vi "Result.Parse STD OUT Text, Create Result Data.vi"(4 "UUTDir":path, 6 "Prefix":string, 7 "Category":string, 8 "Version Name":string, 9 "Error Code":i32, 10 "Task Name":string, 11 "StdOut":string) -> (0 "Error":errorcluster, 1 "SW Ver":T4[](array[typedef]), 2 "Numeric":T5[](array[typedef]) {"Status" items=["LOG", "PASS", "FAIL", "ERROR"]}, 3 "Attr":T2[](array[typedef]) {"Status" items=["LOG", "PASS", "FAIL", "ERROR"]}, 5 "Data Files":T1[](array[typedef]))   [LabVIEW 2018]
uses:
  Result.Numeric.ctl
  Result.Limit Type.ctl
  Result.Measurement and Attribute Item Status.ctl
  Result XML/TestResult.SW Item.ctl
  Result.Attribute.ctl
  Reports/Report.Result FileDataObject.ctl
  Errors/Error.Error Code List.ctl
  <vilib>/KATE/Files/File Utils.lvlib
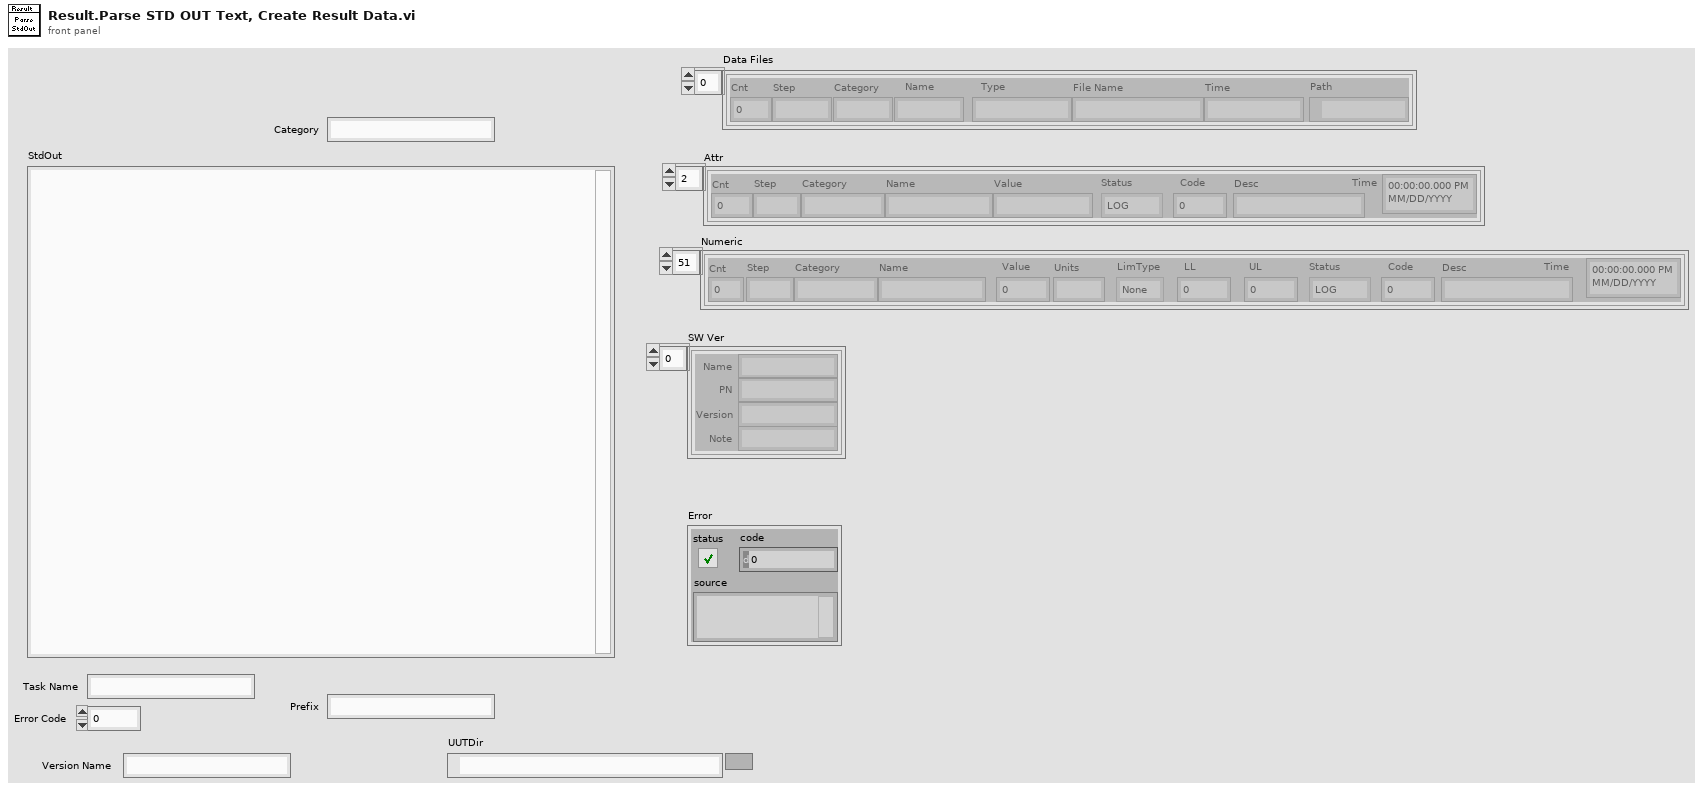
[diagram p1: front panel]
types:
  T1 = typedef "Report.Result FileDataObject.ctl" = cluster{"Cnt":i32, "Step":string, "Category":string, "Name":string, "Type":string, "File Name":string, "Time":string, "Path":path}
  T2 = typedef "Result.Attribute.ctl" = cluster{"Cnt":i32, "Step":string, "Category":string, "Name":string, "Value":string, "Status":T3, "Code":i32, "Desc":string, "Time":timestamp}
  T3 = typedef "Result.Measurement and Attribute Item Status.ctl" = i32
  T4 = typedef "TestResult.SW Item.ctl" = cluster{"Name":string, "PN":string, "Version":string, "Note":string}
  T5 = typedef "Result.Numeric.ctl" = cluster{"Cnt":i32, "Step":string, "Category":string, "Name":string, "Value":dbl, "Units":string, "LimType":T6, "LL":dbl, "UL":dbl, "Status":T3, "Code":i32, "Desc":string, "Time":timestamp}
  T6 = typedef "Result.Limit Type.ctl" = enum16{"None", "EQ", "NE", "GT", "LT", "GE", "LE", "GTLT", "GELE", "GELT", "GTLE", "LTGT", "LEGE", "LEGT", "LTGE", "Contains", "NotContains"}
  T7 = cluster{"Attr":T2[], "Numeric":T5[], "SW Ver":T4[], "Error":errorcluster, "Data Files":T1[]}
  T8 = typedef "Error.Error Code List.ctl" = i32
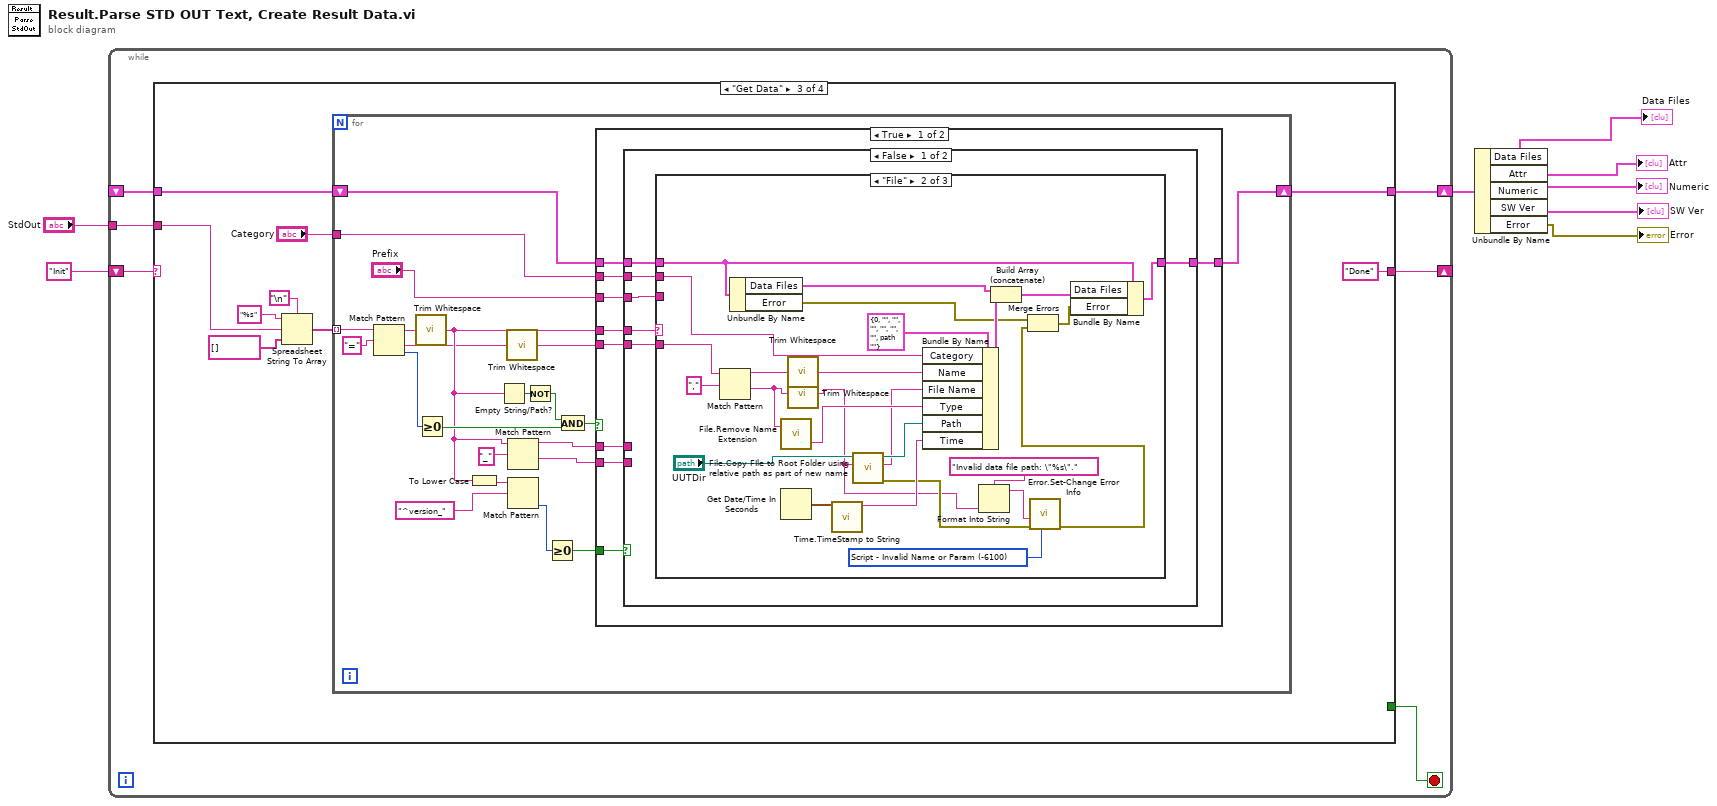
[diagram p0: block diagram]
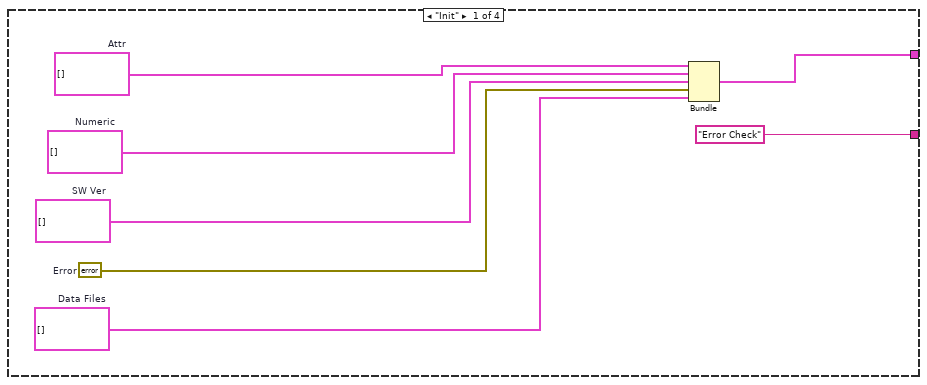
[diagram p2: hidden frame]
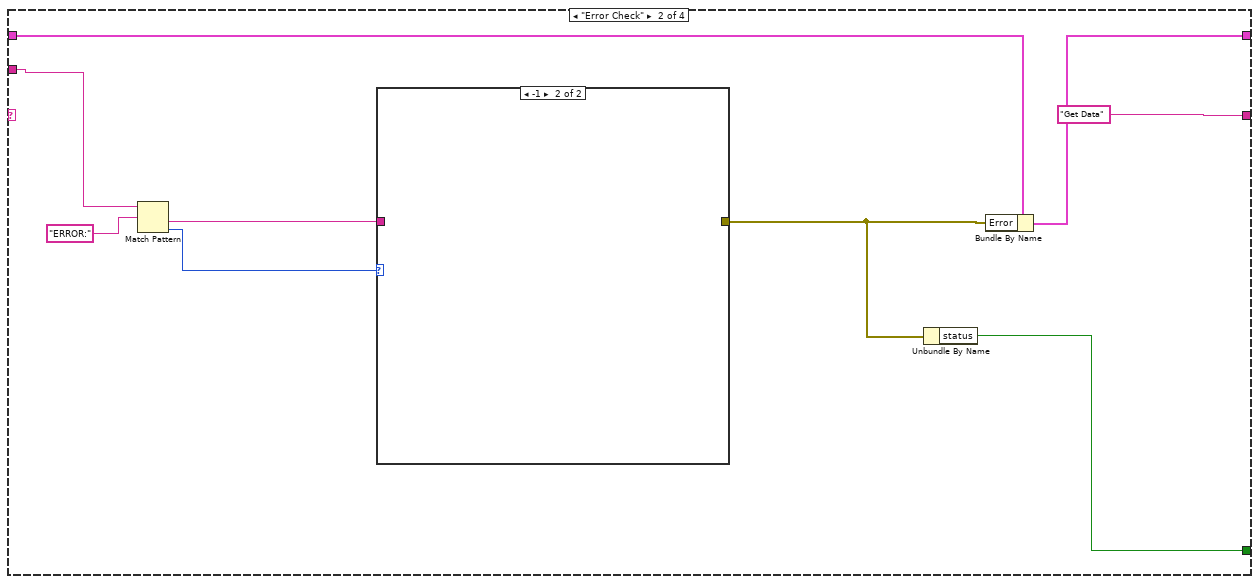
[diagram p3: hidden frame]
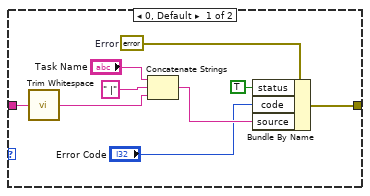
[diagram p4: hidden frame]
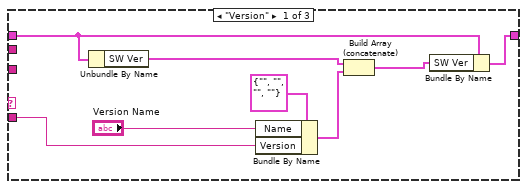
[diagram p5: hidden frame]
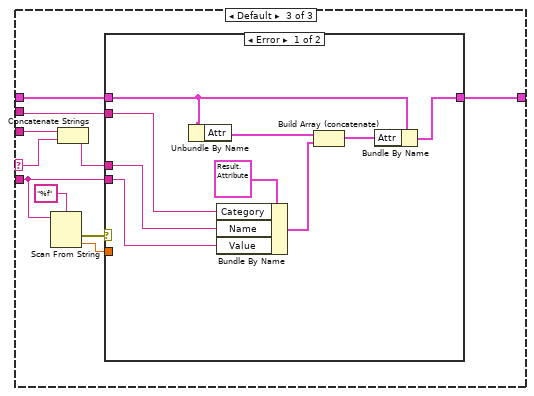
[diagram p6: hidden frame]
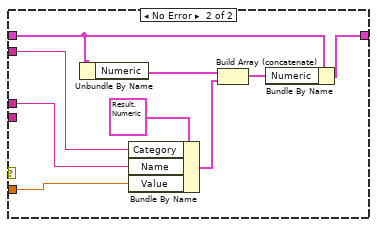
[diagram p7: hidden frame]
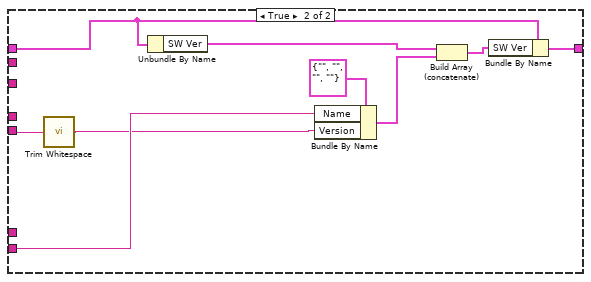
[diagram p8: hidden frame]
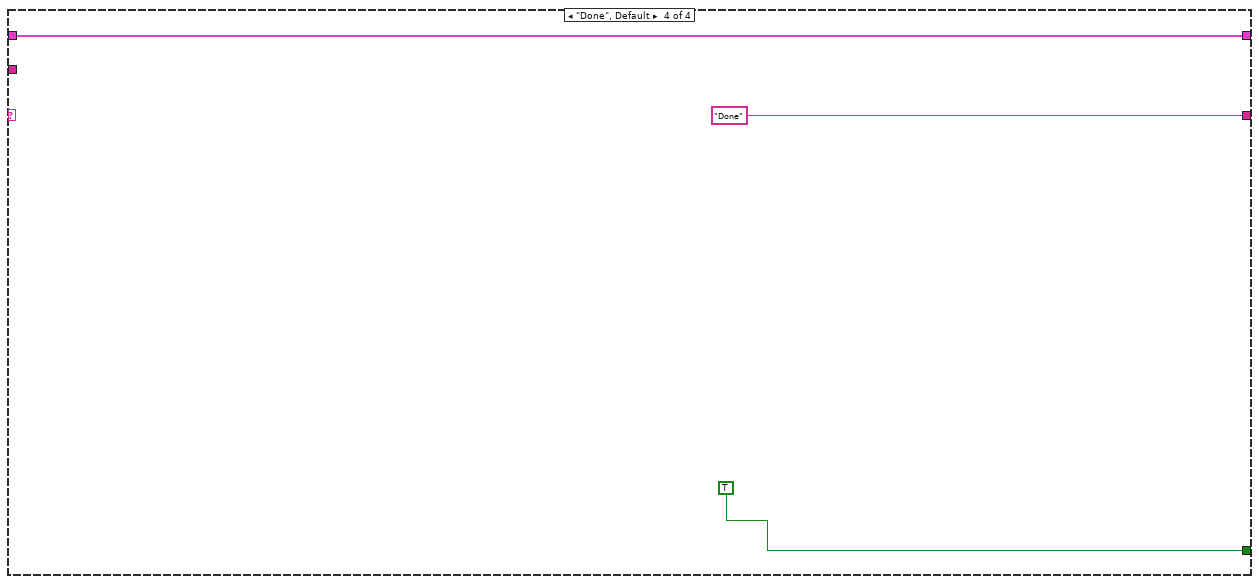
[diagram p10: hidden frame]
diagram:
  n1 = while {
    tunnel: "StdOut" -> [w14]
    shift-right: [w10] -> _
    shift-left: "Init" -> [w13]
    shift-right: [w11] -> w6
    shift-left: _ -> [w12]
    stop <- w9 stop-if-true
    n2 = case shown="\"Get Data\"" w13 {
      tunnel: w14 -> [_ w26 w45 _]
      tunnel: w12 -> [_ w29 w42 w158]
      tunnel: [w18 w28 w40 w158] -> w11
      tunnel: ["Error Check" "Get Data" "Done" "Done"] -> w10
      tunnel: [_ w22 _ TRUE] -> w9
      frame "Init" {
        w15 = T1[] []  # Data Files
        w16 = errorcluster {"status"=FALSE, "code"=0, "source"=""}  # Error
        w20 = T5[] []  # Numeric
        w21 = T2[] []  # Attr
        w19 = T4[] []  # SW Ver
        n3 = Bundle("Attr"=w21, "Numeric"=w20, "SW Ver"=w19, "Error"=w16, "Data Files"=w15) -> (w18:T7)  [unwired: 1 in]
      }
      frame "Error Check" {
        n4 = Match Pattern(string=w26, regular expression="ERROR:") -> (after substring=w25:string, offset past match=w24:i32)  [unwired: 1 in, 2 out]
        n5 = case shown="-1" w24 {
          tunnel: w25 -> [w39 _]
          tunnel: [w31 _] -> w23
          frame 0, Default {
            w38 = errorcluster {"status"=FALSE, "code"=0, "source"=""}  # Error
            n6 = call <vilib>:"Trim Whitespace.vi"("string"=w39) -> ("trimmed string"=w36:string)  [unwired: 1 in]
            n7 = Concatenate Strings("Task Name", " |", w36) -> (w33:string)
            n8 = Bundle By Name(cluster=w38, "status"=TRUE, "code"="Error Code", "source"=w33) -> (w31:errorcluster)
          }
          frame -1 {
          }
        }
        n9 = Unbundle By Name(w23) -> ("status"=w22:bool)
        n10 = Bundle By Name(cluster=w29, "Error"=w23) -> (w28:T7)
      }
      frame "Get Data" {
        n11 = Spreadsheet String To Array(delimiter (Tab)="\n", format string="%s" ("spreadsheet string"), spreadsheet string=w45, array type (2D Dbl)=string[] []) -> (array=w43:string[])
        n12 = for {
          tunnel: w43 -> [w70] mode=indexing
          shift-right: [w67] -> w40
          shift-left: w42 -> [w68]
          tunnel: "Category" -> [w60]
          n13 = Match Pattern(string=w70, regular expression="=") -> (before substring=w66:string, after substring=w50:string, offset past match=w65:i32)  [unwired: 1 in, 1 out]
          n14 = call <vilib>:"Trim Whitespace.vi"("string"=w66) -> ("trimmed string"=w51:string)  [unwired: 1 in]
          n15 = Greater Or Equal To 0?(x=w65) -> (x >= 0?=w62:bool)
          n16 = To Lower Case(string=w51) -> (all lower case string=w55:string)
          n17 = Empty String/Path?(string/path=w51) -> (empty?=w64:bool)
          n18 = call <vilib>:"Trim Whitespace.vi"("string"=w50) -> ("trimmed string"=w49:string)  [unwired: 1 in]
          n19 = Match Pattern(string=w51, regular expression="_") -> (before substring=w54:string, after substring=w53:string)  [unwired: 1 in, 2 out]
          n20 = Match Pattern(string=w55, regular expression="^version_") -> (offset past match=w58:i32)  [unwired: 1 in, 3 out]
          n21 = Not(x=w64) -> (.not. x?=w63:bool)
          n22 = Greater Or Equal To 0?(x=w58) -> (x >= 0?=w57:bool)
          n23 = And(x=w63, y=w62) -> (x .and. y?=w61:bool)
          n24 = case shown="True" w61 {
            tunnel: w68 -> [w77 w157]
            tunnel: [w76 w157] -> w67
            tunnel: w49 -> [w79 _]
            tunnel: w51 -> [w75 _]
            tunnel: w60 -> [w78 _]
            tunnel: "Prefix" -> [w74 _]
            tunnel: w54 -> [w71 _]
            tunnel: w53 -> [w72 _]
            tunnel: w57 -> [w73 _]
            frame True {
              n25 = case shown="False" w73 {
                tunnel: w79 -> [w85 w149]
                tunnel: w78 -> [w84 _]
                tunnel: w77 -> [w83 w151]
                tunnel: [w82 w152] -> w76
                tunnel: w75 -> [w81 _]
                tunnel: w74 -> [w80 _]
                tunnel: w72 -> [_ w150]
                tunnel: w71 -> [_ _]
                frame False {
                  n26 = case shown="\"File\"" w81 {
                    selector: w81 -> [_ _ w121]
                    tunnel: w85 -> [w86 w106 w126]
                    tunnel: w84 -> [_ w113 w122]
                    tunnel: w83 -> [w92 w102 w125]
                    tunnel: [w91 w119 w124] -> w82
                    tunnel: w80 -> [_ _ w123]
                    frame "Version" {
                      n27 = Unbundle By Name(w92) -> ("SW Ver"=w89:T4[])
                      n28 = Bundle By Name(cluster=T4 {"Name"="", "PN"="", "Version"="", "Note"=""} ("SW_Item"), "Name"="Version Name", "Version"=w86) -> (w88:T4)
                      n29 = Build Array (concatenate)(w89, w88) -> (w90:T4[])
                      n30 = Bundle By Name(cluster=w92, "SW Ver"=w90) -> (w91:T7)
                    }
                    frame "File" {
                      w98 = T8 -6100 items=["No Error"=0, "Abort"=-2, "Misc"=-5000, "Fixture Error"=-5100, "File IO - General"=-5200, "FIle IO - Config Error"=-5201, "Instrument - General"=-5300, "Instrument - Serial Com"=-5301, "Instrument - Camera"=-5302, "Instrument - PS"=-5303, "Instrument - Oscilloscope"=-5304, "Instrument - Function Gen"=-5305, "Instrument - Load"=-5306, "Instrument - Meter"=-5307, "Instrument - Power Control"=-5308, "Instrument - Motion"=-5309, "Instrument - RF"=-5310, "System Exe"=-5400, "Image Processing"=-5500, "Communication"=-5600, "Script - Syntax Error"=-6000, "Script - Invalid Name or Param"=-6100, "Script - Timeout"=-6200, "Invalid Data"=-6300, "FW Update Error"=-6500] ("Std Code")
                      n31 = Match Pattern(string=w106, regular expression=",") -> (before substring=w111:string, after substring=w109:string)  [unwired: 1 in, 2 out]
                      n32 = Unbundle By Name(w102) -> ("Data Files"=w117:T1[], "Error"=w100:errorcluster)
                      n33 = call <vilib>:"File.Remove Name Extension.vi"("File Name"=w109) -> ("Ext"=w110:string)  [unwired: 1 in, 1 out]
                      n34 = Get Date/Time In Seconds() -> (seconds since 1Jan1904=w108:timestamp)
                      n35 = call <vilib>:"Trim Whitespace.vi"("string"=w111) -> ("trimmed string"=w112:string)  [unwired: 1 in]
                      n36 = call <vilib>:"Trim Whitespace.vi"("string"=w109) -> ("trimmed string"=w95:string)  [unwired: 1 in]
                      n37 = call "Time.TimeStamp to String.vi"("Time Stamp in"=w108) -> ("Time String Out"=w107:string)  [unwired: 10 in]
                      n38 = call "File.Copy FIle to Root Folder using relative path as part of new name.vi"("Relative Path"=w95, "Root Path"="UUTDir") -> ("error out"=w99:errorcluster, "New File Name"=w103:string, "Adjusted Path"=w104:path)  [unwired: 6 in, 1 out]
                      n39 = Bundle By Name(cluster=T1 {"Cnt"=0, "Step"="", "Category"="", "Name"="", "Type"="", "File Name"="", "Time"="", "Path"=path ""} ("FileData Object"), "Category"=w113, "Name"=w112, "File Name"=w103, "Type"=w110, "Path"=w104, "Time"=w107) -> (w116:T1)
                      n40 = Format Into String(format string="Invalid data file path: \"%s\".", w95) -> (resulting string=w96:string)  [unwired: 2 in, 1 out]
                      n41 = Build Array (concatenate)(w117, w116) -> (w118:T1[])
                      n42 = call "Error.Set-Change Error Info.vi"("Std Code"=w98, "error in"=w99, "Description"=w96) -> ("error out"=w94:errorcluster)  [unwired: 8 in]
                      n43 = Merge Errors(w100, w94) -> (w101:errorcluster)
                      n44 = Bundle By Name(cluster=w102, "Data Files"=w118, "Error"=w101) -> (w119:T7)
                    }
                    frame Default {
                      n45 = Scan From String(format string="%f", input string=w126) -> (error out=w128:errorcluster, output 1=w127:dbl)  [unwired: 3 in, 2 out]
                      n46 = Concatenate Strings(w123, w121) -> (w120:string)
                      n47 = case shown="Error" w128 {
                        tunnel: w127 -> [_ w140]
                        tunnel: w120 -> [w136 w139]
                        tunnel: w126 -> [w137 _]
                        tunnel: w122 -> [w135 w147]
                        tunnel: w125 -> [w132 w144]
                        tunnel: [w130 w142] -> w124
                        frame Error {
                          n48 = Unbundle By Name(w132) -> ("Attr"=w134:T2[])
                          n49 = Bundle By Name(cluster=T2 {"Cnt"=0, "Step"="", "Category"="", "Name"="", "Value"="", "Status"=0, "Code"=0, "Desc"="", "Time"=timestamp(0 s since 1904-01-01)} ("Attribute"), "Category"=w135, "Name"=w136, "Value"=w137) -> (w133:T2)
                          n50 = Build Array (concatenate)(w134, w133) -> (w131:T2[])
                          n51 = Bundle By Name(cluster=w132, "Attr"=w131) -> (w130:T7)
                        }
                        frame No Error {
                          n52 = Unbundle By Name(w144) -> ("Numeric"=w146:T5[])
                          n53 = Bundle By Name(cluster=T5 {"Cnt"=0, "Step"="", "Category"="", "Name"="", "Value"=0.0, "Units"="", "LimType"=enum."None", "LL"=0.0, "UL"=0.0, "Status"=0, "Code"=0, "Desc"="", "Time"=timestamp(0 s since 1904-01-01)} ("Measurement"), "Category"=w147, "Name"=w139, "Value"=w140) -> (w145:T5)
                          n54 = Build Array (concatenate)(w146, w145) -> (w143:T5[])
                          n55 = Bundle By Name(cluster=w144, "Numeric"=w143) -> (w142:T7)
                        }
                      }
                    }
                  }
                }
                frame True {
                  n56 = call <vilib>:"Trim Whitespace.vi"("string"=w149) -> ("trimmed string"=w148:string)  [unwired: 1 in]
                  n57 = Unbundle By Name(w151) -> ("SW Ver"=w154:T4[])
                  n58 = Bundle By Name(cluster=T4 {"Name"="", "PN"="", "Version"="", "Note"=""} ("SW_Item"), "Name"=w150, "Version"=w148) -> (w153:T4)
                  n59 = Build Array (concatenate)(w154, w153) -> (w155:T4[])
                  n60 = Bundle By Name(cluster=w151, "SW Ver"=w155) -> (w152:T7)
                }
              }
            }
            frame False {
            }
          }
        }
      }
      frame "Done", Default {
      }
    }
  }
  n61 = Unbundle By Name(w6) -> ("Data Files"=→"Data Files":T1[], "Attr"=→"Attr":T2[], "Numeric"=→"Numeric":T5[], "SW Ver"=→"SW Ver":T4[], "Error"=→"Error":errorcluster)
